vi "Tag Set__icon_lib_labview_project_api.vi"(6 "Is Persistent":bool, 8 "error in (no error)":errorcluster, 9 "Value":variant, 10 "Tag Name":string, 11 "Build Spec Reference":refnum<vi>) -> (0 "error out":errorcluster, 3 "Build Spec Reference Dup":refnum<vi>)   [LabVIEW 2016, in "LabVIEW Project API__icon_lib_labview_project_api.lvlib"]
doc: "Set's a Project Tag's Value\n\n<b>Author:</b> JG\n\n<b>ICON Technologies Pty Ltd</b>\nCopyright (C) 1990-2009\nAll Rights Reserved"
uses:
  LabVIEW Project API__icon_lib_labview_project_api.lvlib
panel:
  # "Output"
  # "Input"
  # "ICON Technologies Pty Ltd\nCopyright (C) 1990-2009\nAll Rights Reserved"
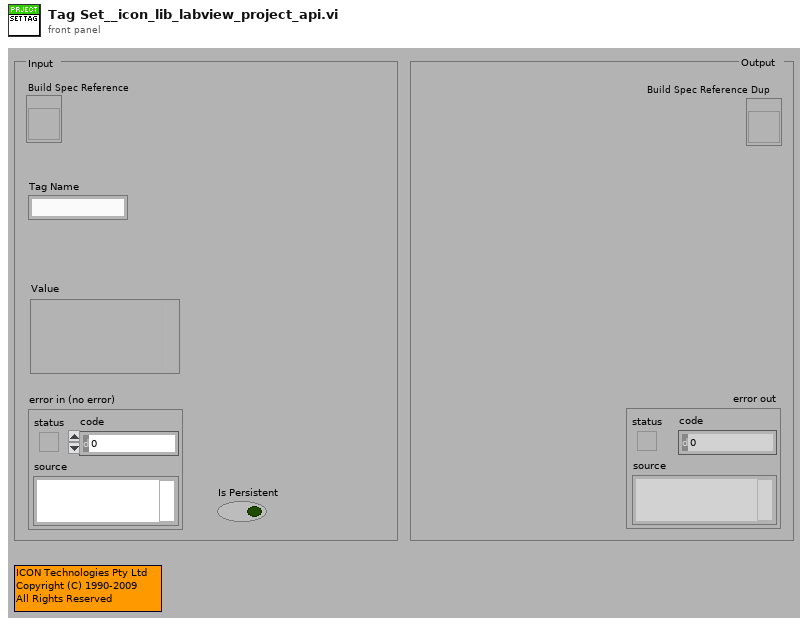
[diagram p1: front panel]
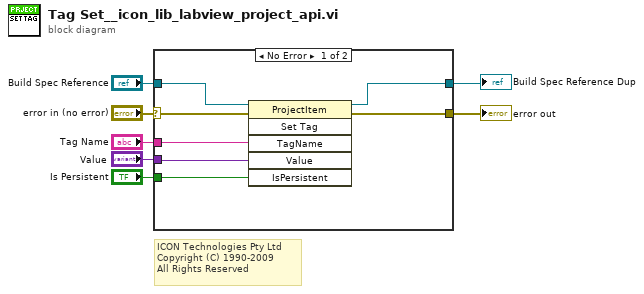
[diagram p0: block diagram]
diagram:
  # "ICON Technologies Pty Ltd\nCopyright (C) 1990-2009\nAll Rights Reserved"
  n1 = case shown="No Error" "error in (no error)" {
    selector: "error in (no error)" -> [w12 w16]
    tunnel: [w14 w16] -> w6
    tunnel: "Build Spec Reference" -> [w13 w15]
    tunnel: [w11 w15] -> w4
    tunnel: "Value" -> [w9 _]
    tunnel: "Tag Name" -> [w10 _]
    tunnel: "Is Persistent" -> [w8 _]
    frame No Error {
      n2 = invoke class="ProjectItem" method="Set Tag"(reference=w13, error in=w12, "TagName"=w10, "Value"=w9, "IsPersistent"=w8) -> (reference out=w11:refnum<vi>, error out=w14:errorcluster)  [unwired: 1 in, 4 out]
    }
    frame Error {
    }
  }
  "error out" <- w6
  "Build Spec Reference Dup" <- w4
